vi "NumericArrayToDotMatrix.vi"(1 "NumericArray":dbl[][](array[numeric]), 2 "Intensity Threshold":i32(knob)=200 scale=0.0..255.0, 3 "Invert Image":bool) -> (0 "DotMatrix":bool[][](array[boolean]))   [LabVIEW 2018]
panel:
  # "Inputs"
  # "Outputs"
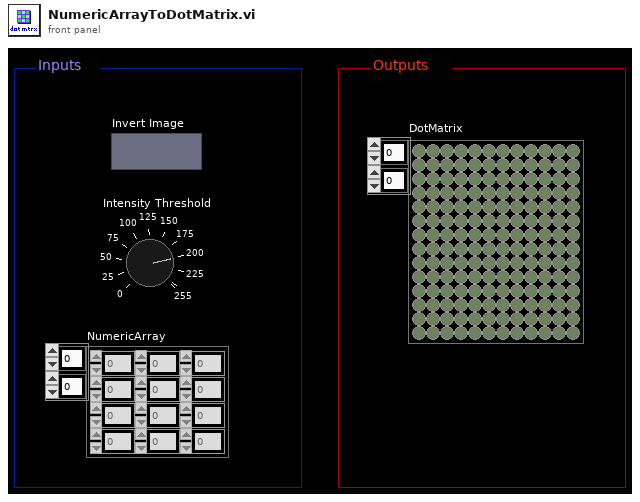
[diagram p1: front panel]
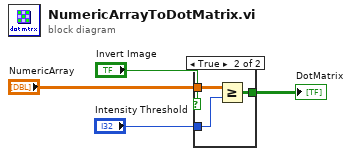
[diagram p0: block diagram]
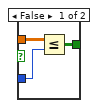
[diagram p2: hidden frame]
diagram:
  n1 = case shown="True" "Invert Image" {
    tunnel: "NumericArray" -> [w7 w10]
    tunnel: [w5 w9] -> w2
    tunnel: "Intensity Threshold" -> [w6 w8]
    frame False {
      n2 = Less Or Equal?(x=w7, y=w6) -> (x <= y?=w5:bool[][])
    }
    frame True {
      n3 = Greater Or Equal?(x=w10, y=w8) -> (x >= y?=w9:bool[][])
    }
  }
  "DotMatrix" <- w2
